vi "Fission Reactor.vi"(8 "Activate":bool, 9 "Burn Rate (mB/t)":dbl, 11 "Build Specifications":T1={"Length (m)"=3, "Width (m)"=3, "Height (m)"=4, "Coolant Type"=enum."Water"} {"Height (m)" min=4 max=18 step=1; "Width (m)" min=3 max=18 step=1; "Length (m)" min=3 max=18 step=1}) -> (1 "Theoretical Heating Rate (mB/t)":u32, 2 "Actual Burn Rate (mB/t)":dbl(knob) scale=0.0..1920.0, 3 "Computed Build Properties":T2)   [LabVIEW 2026]
uses:
  Fission Reactor Build Properties.ctl
  Fission Reactor Build Specifications.ctl
panel:
  # "Fission Reactor Design"
  # "Fission Reactor Control"
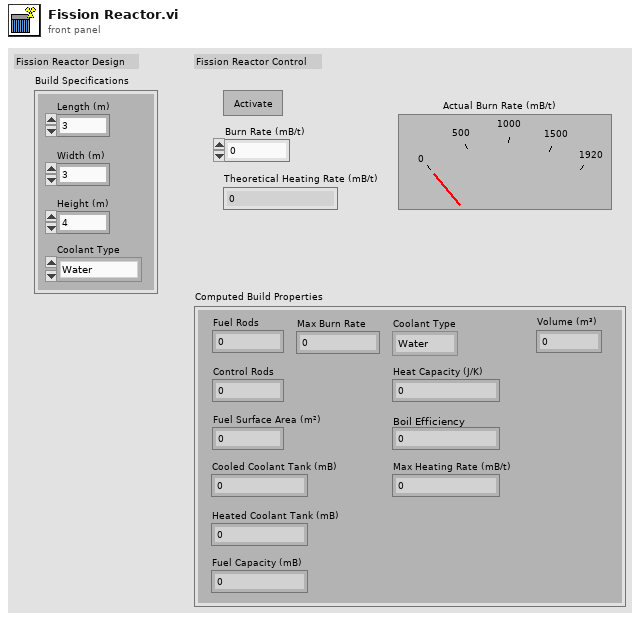
[diagram p1: front panel]
types:
  T1 = typedef "Fission Reactor Build Specifications.ctl" = cluster{"Length (m)":i32, "Width (m)":i32, "Height (m)":i32, "Coolant Type":enum16{"Water", "Sodium"}}
  T2 = typedef "Fission Reactor Build Properties.ctl" = cluster{"Fuel Rods":i32, "Control Rods":i32, "Volume (m³)":i32, "Fuel Surface Area (m²)":i32, "Cooled Coolant Tank (mB)":i32, "Fuel Capacity (mB)":i64, "Heat Capacity (J/K)":dbl, "Max Burn Rate":i64, "Max Heating Rate (mB/t)":i64, "Boil Efficiency":dbl, "Coolant Type":enum16{"Water", "Sodium"}, "Heated Coolant Tank (mB)":i64}
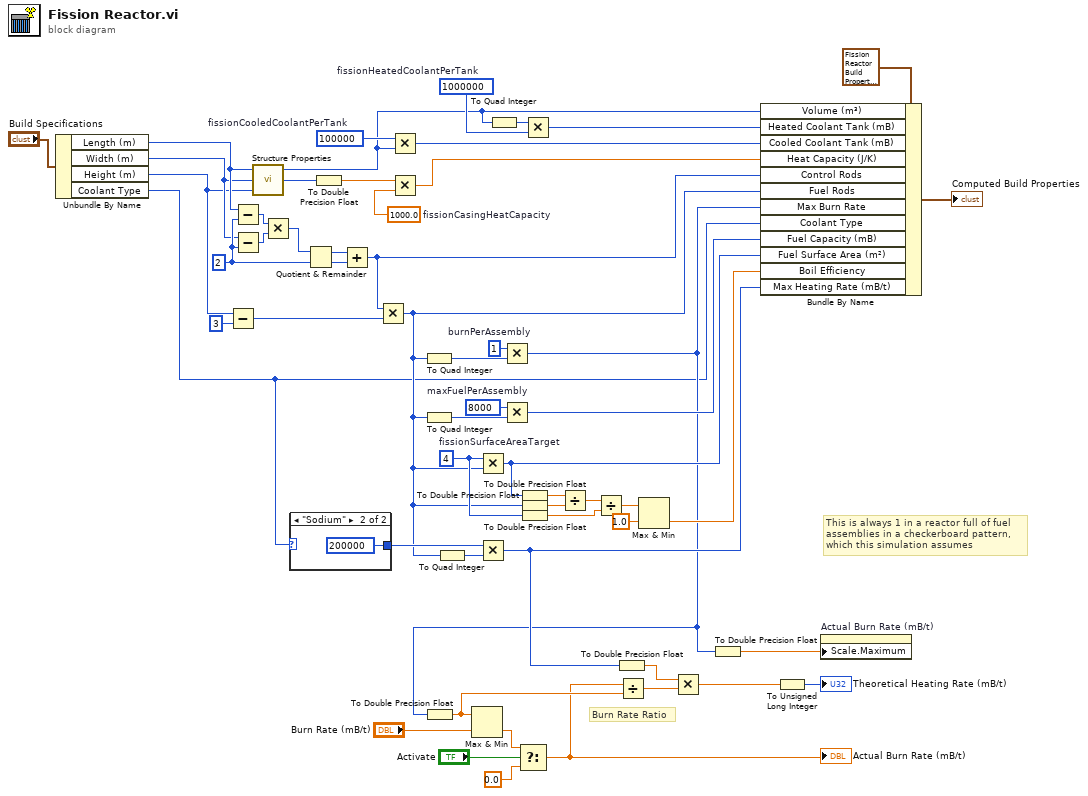
[diagram p0: block diagram]
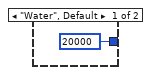
[diagram p2: hidden frame]
diagram:
  w9 = i64 1  # burnPerAssembly
  w18 = i64 1000000  # fissionHeatedCoolantPerTank
  w45 = 1000.0  # fissionCasingHeatCapacity
  w13 = 4  # fissionSurfaceAreaTarget
  w48 = i64 8000  # maxFuelPerAssembly
  w47 = 100000  # fissionCooledCoolantPerTank
  w38 = 2 ("y")
  # "This is always 1 in a reactor full of fuel\nassemblies in a checkerboard pattern,\nwhich this simulation assumes"
  # "Burn Rate Ratio"
  n1 = Unbundle By Name("Build Specifications") -> ("Length (m)"=w5:i32, "Width (m)"=w4:i32, "Height (m)"=w3:i32, "Coolant Type"=w2:enum16{"Water", "Sodium"})
  n2 = Subtract(x=w3, y=3) -> (x-y=w55:i32)
  n3 = Subtract(x=w5, y=w38) -> (x-y=w37:i32)
  n4 = Subtract(x=w4, y=w38) -> (x-y=w36:i32)
  n5 = call "Structure Properties.vi"("Length"=w5, "Width"=w4, "Height"=w3) -> ("Volume"=w17:i32, "Casing"=w46:i32)  [unwired: 2 in, 3 out]
  n6 = Multiply(x=w37, y=w36) -> (x*y=w35:i32)
  n7 = case shown="\"Sodium\"" w2 {
    tunnel: [i64 20000 ("x") i64 200000 ("x")] -> w22
    frame "Water", Default {
    }
    frame "Sodium" {
    }
  }
  n8 = Quotient & Remainder(x=w35, y=w38) -> (x-y*floor(x/y)=w54:i32, floor(x/y)=w53:i32)
  n9 = To Double Precision Float(number=w46) -> (double precision float=w21:dbl)
  n10 = Add(x=w54, y=w53) -> (x+y=w32:i32)
  n11 = Multiply(x=w32, y=w55) -> (x*y=w8:i32)
  n12 = Multiply(x=w47, y=w17) -> (x*y=w34:i32)
  n13 = Multiply(x=w21, y=w45) -> (x*y=w33:dbl)
  n14 = To Quad Integer(1:w8) -> (0:w10:i64)
  n15 = To Quad Integer(1:w8) -> (0:w14:i64)
  n16 = To Quad Integer(1:w8) -> (0:w11:i64)
  n17 = Multiply(x=w13, y=w8) -> (x*y=w29:i32)
  n18 = Multiply(x=w22, y=w11) -> (x*y=w20:i64)
  n19 = To Quad Integer(1:w17) -> (0:w16:i64)
  n20 = Multiply(x=w9, y=w10) -> (x*y=w7:i64)
  n21 = To Double Precision Float(number=w7) -> (double precision float=w43:dbl)
  n22 = Max & Min(x=w43, y="Burn Rate (mB/t)") -> (min(x,y)=w44:dbl)  [unwired: 1 out]
  n23 = Multiply(x=w48, y=w14) -> (x*y=w15:i64)
  n24 = Select(t=w44, s="Activate", f=0.0) -> (s? t:f=w6:dbl)
  "Actual Burn Rate (mB/t)" <- w6
  n25 = To Double Precision Float(number=w29) -> (double precision float=w28:dbl)
  n26 = To Double Precision Float(number=w8) -> (double precision float=w27:dbl)
  n27 = To Double Precision Float(number=w13) -> (double precision float=w12:dbl)
  n28 = Multiply(x=w16, y=w18) -> (x*y=w19:i64)
  n29 = Divide(x=w28, y=w27) -> (x/y=w26:dbl)
  n30 = Divide(x=w26, y=w12) -> (x/y=w24:dbl)
  n31 = To Double Precision Float(number=w20) -> (double precision float=w39:dbl)
  n32 = Divide(x=w6, y=w43) -> (x/y=w42:dbl)
  n33 = Max & Min(x=w24, y=1.0) -> (min(x,y)=w25:dbl)  [unwired: 1 out]
  n34 = Multiply(x=w39, y=w42) -> (x*y=w41:dbl)
  n35 = To Double Precision Float(number=w7) -> (double precision float=w52:dbl)
  n36 = Bundle By Name(cluster=T2 {"Fuel Rods"=0, "Control Rods"=0, "Volume (m³)"=0, "Fuel Surface Area (m²)"=0, "Cooled Coolant Tank (mB)"=0, "Fuel Capacity (mB)"=0, "Heat Capacity (J/K)"=0.0, "Max Burn Rate"=0, "Max Heating Rate (mB/t)"=0, "Boil Efficiency"=0.0, "Coolant Type"=enum."Water", "Heated Coolant Tank (mB)"=0} ("Reactor Build Properties"), "Volume (m³)"=w17, "Heated Coolant Tank (mB)"=w19, "Cooled Coolant Tank (mB)"=w34, "Heat Capacity (J/K)"=w33, "Control Rods"=w32, "Fuel Rods"=w8, "Max Burn Rate"=w7, "Coolant Type"=w2, "Fuel Capacity (mB)"=w15, "Fuel Surface Area (m²)"=w29, "Boil Efficiency"=w25, "Max Heating Rate (mB/t)"=w20) -> (→"Computed Build Properties":T2)
  n37 = To Unsigned Long Integer(number=w41) -> (unsigned 32bit integer=→"Theoretical Heating Rate (mB/t)":u32)
  n38 = property on="Actual Burn Rate (mB/t)" class="Knob (strict)"("Scale.Maximum"=w52) -> ()  [unwired: 2 in, 2 out]
